vi "GET_volume_last_update.vi"(8 "error in (no error)":errorcluster, 10 "volume id":string="4050-75888", 11 "REST Client in":refnum<class "REST Client.lvclass">) -> (0 "error out":errorcluster, 2 "results.date_last_updated":timestamp, 3 "REST Client out":refnum<class "REST Client.lvclass">)   [LabVIEW 2024, in "CV_RESTful_Lib.lvlib"]
uses:
  CV_RESTful_Lib.lvlib
  <vilib>/addons/_JKI.lib/REST Client/classes/REST Client/REST Client.lvclass
  <vilib>/addons/_JKI.lib/REST Client/classes/REST Client/HTTP Header.ctl
  <vilib>/NI/Advanced HTTP Client/Header--Combo Box.ctl
  <vilib>/NI/Advanced HTTP Client/Session.lvclass
  <vilib>/addons/_JKI.lib/Serialization/JSON/JKI JSON Serialization.lvlib
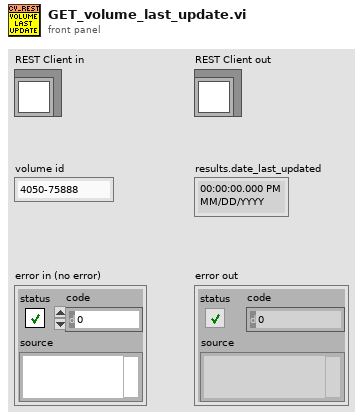
[diagram p1: front panel]
types:
  T1 = cluster{"status_code":i32, "results":cluster{"date_last_updated":timestamp}}
  T2 = typedef "REST Client.lvlib/REST Client.lvclass/HTTP Header.ctl" = cluster{"header":T3, "value":string}
  T3 = typedef "lib_NI_Advanced HTTP Client.lvlib/Session.lvclass/Header--Combo Box.ctl" = string
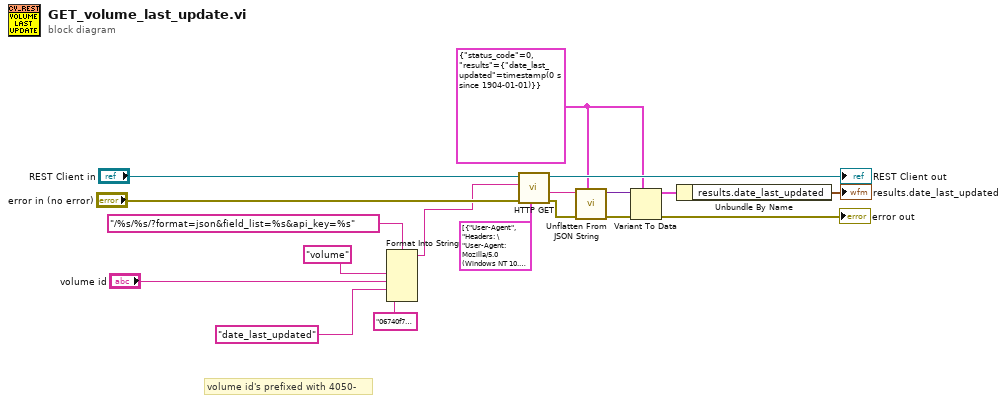
[diagram p0: block diagram]
diagram:
  w3 = T1 {"status_code"=0, "results"={"date_last_updated"=timestamp(0 s since 1904-01-01)}}
  # "volume id's prefixed with 4050-"
  n1 = Format Into String(format string="/%s/%s/?format=json&field_list=%s&api_key=%s", "volume" ("resource"), "volume id", "date_last_updated" ("String"), "06740f73403e0b211d597c50ea94c7f16ea5e8ea") -> (resulting string=w13:string)  [unwired: 2 in, 1 out]
  n2 = call-dynamic "HTTP GET.vi"("request specific headers"=T2[] [{"header"="User-Agent", "value"="Headers: \"User-Agent: Mozilla/5.0 (Windows NT 10.0; Win64; x64) AppleWebKit/537.36 (KHTML, like Gecko) Chrome/91.0.4472.101 Safari/537.36\""}], "error in (no error)"="error in (no error)", "Path"=w13, "REST Client in"="REST Client in") -> ("error out"=w18:errorcluster, "Response body"=w10:string, "REST Client out"=→"REST Client out":refnum<class "REST Client.lvclass">)  [unwired: 2 in, 3 out]
  n3 = call <vilib>:"Unflatten From JSON String.vi"("Type and Defaults"=w3, "error in"=w18, "JSON String"=w10) -> ("error out"=w8:errorcluster, "Variant"=w9:variant)  [unwired: 7 in]
  n4 = Variant To Data(error in=w8, type=w3, Variant=w9) -> (data=w2:T1, error out=→"error out":errorcluster)
  n5 = Unbundle By Name(w2) -> ("results.date_last_updated"=→"results.date_last_updated":timestamp)
